vi "Get Config Variables.vi"(8 "error in (no error)":errorcluster, 10 "ReadBufferView":i32, 11 "LabVIEW Web Service Request":refnum<class "Web Request.lvclass">) -> (0 "error out":errorcluster, 3 "LabVIEW Web Service Request out":refnum<class "Web Request.lvclass">)   [LabVIEW 2018]
doc: "This VI sets all of the ESP variables for a single contact so it can be output from an ESP script."
uses:
  <vilib>/wsapi/Web Request.lvclass
  subvis/i32 to dec string small.vi
  CAEN globals.vi
  subvis/dbl to fr string small.vi
  <vilib>/wsapi/class/subVIs/Set Many String ESP Variables.vi
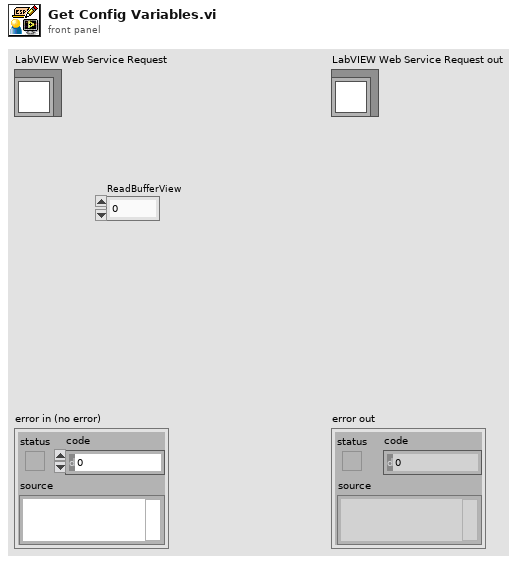
[diagram p1: front panel]
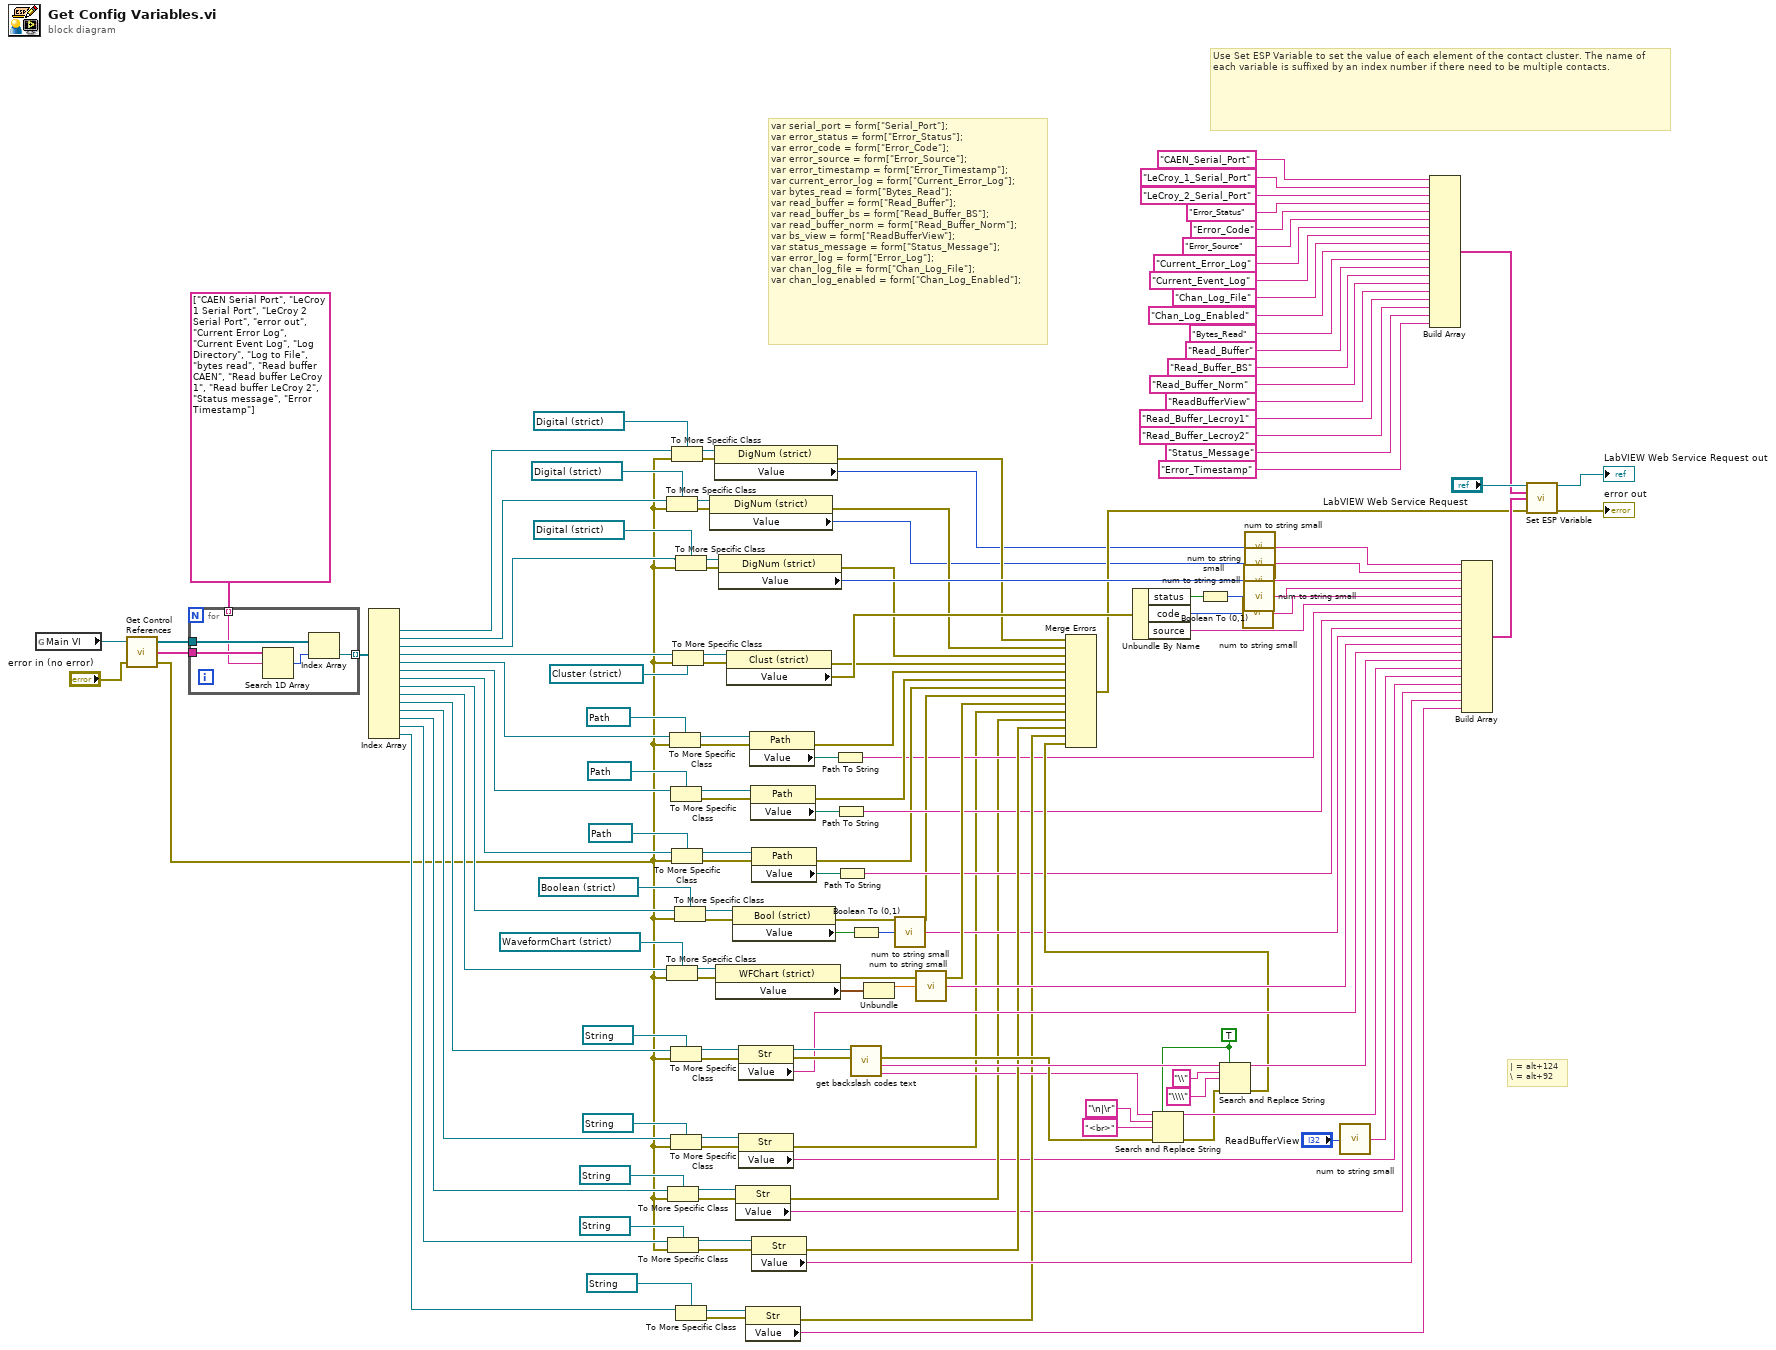
[diagram p0: block diagram]
diagram:
  w66 = TRUE ("replace all? (F)")
  # "| = alt+124\n\\ = alt+92"
  # "var serial_port = form[\"Serial_Port\"];\nvar error_status = form[\"Error_Status\"];\nvar error_code = form[\"Error_Code\"];\nvar error_source = form[\"Error_Source\"];\nvar error_timestamp = form[\"Error_Timestamp\"];\nvar current_error_log = form[\"Current_Error_Log\"];\nvar bytes_read = form[\"Bytes_Read\"];\nvar read_buffer = form[\"Read_Buffer\"];\nvar read_buffer_bs = form[\"Read_Buffer_BS\"];\nvar read_buffer_norm = form[\"Read_Buffer_Norm\"];\nvar bs_view = form[\"ReadBufferView\"];\nvar status_message = form[\"Status_Message\"];\nvar error_log = form[\"Error_Log\"];\nvar chan_log_file = form[\"Chan_Log_File\"];\nvar chan_log_enabled = form[\"Chan_Log_Enabled\"];"
  # "Use Set ESP Variable to set the value of each element of the contact cluster. The name of each variable is suffixed by an index number if there need to be multiple contacts."
  n1 = global read "CAEN globals.vi" "Main VI"() -> (w134:refnum<vi>)
  n2 = call "Get Control References.vi"("error in"="error in (no error)", "This vi"=w134) -> ("error out"=w3:errorcluster, "Control Names"=w133:string[], "Controls[]"=w132:refnum<vi>[])  [unwired: 1 in]
  n3 = for {
    tunnel: w133 -> [w152]
    tunnel: w132 -> [w150]
    tunnel: [w149] -> w124 mode=indexing
    tunnel: string[] ["CAEN Serial Port", "LeCroy 1 Serial Port", "LeCroy 2 Serial Port", "error out", "Current Error Log", "Current Event Log", "Log Directory", "Log to File", "bytes read", "Read buffer CAEN", "Read buffer LeCroy 1", "Read buffer LeCroy 2", "Status message", "Error Timestamp"] ("Control Names") -> [w148] mode=indexing
    n4 = Search 1D Array(1D array=w152, element=w148) -> (index of element=w151:i32)  [unwired: 1 in]
    n5 = Index Array(array=w150, index=w151) -> (element=w149:refnum<vi>)
  }
  n6 = Index Array(array=w124) -> (element #1=w18:refnum<vi>, element #2=w19:refnum<vi>, element #3=w122:refnum<vi>, element #4=w116:refnum<vi>, element #5=w112:refnum<vi>, element #6=w51:refnum<vi>, element #7=w44:refnum<vi>, element #8=w40:refnum<vi>, element #9=w38:refnum<vi>, element #10=w37:refnum<vi>, element #11=w4:refnum<vi>, element #12=w5:refnum<vi>, element #13=w6:refnum<vi>, element #14=w7:refnum<vi>)  [unwired: 14 in]
  n7 = To More Specific Class(target class=refnum<vi> refnum ("code"), reference=w19, error in=w3) -> (specific class reference=w30:refnum<vi>, error out=w29:errorcluster)
  n8 = To More Specific Class(target class=refnum<vi> refnum ("bytes read 2"), reference=w38, error in=w3) -> (specific class reference=w104:refnum<vi>, error out=w103:errorcluster)
  n9 = To More Specific Class(target class=refnum<vi> refnum ("Label.Text"), reference=w5, error in=w3) -> (specific class reference=w13:refnum<vi>, error out=w14:errorcluster)
  n10 = To More Specific Class(target class=refnum<vi> refnum ("Label.Text"), reference=w6, error in=w3) -> (specific class reference=w97:refnum<vi>, error out=w96:errorcluster)
  n11 = To More Specific Class(target class=refnum<vi> refnum ("Error Log Directory"), reference=w112, error in=w3) -> (specific class reference=w109:refnum<vi>, error out=w110:errorcluster)
  n12 = To More Specific Class(target class=refnum<vi> refnum ("Error Log Directory"), reference=w51) -> (specific class reference=w55:refnum<vi>, error out=w54:errorcluster)  [unwired: 1 in]
  n13 = To More Specific Class(target class=refnum<vi> refnum ("Label.Text"), reference=w37, error in=w3) -> (specific class reference=w106:refnum<vi>, error out=w107:errorcluster)
  n14 = To More Specific Class(target class=refnum<vi> refnum ("Label.Text"), reference=w4, error in=w3) -> (specific class reference=w16:refnum<vi>, error out=w15:errorcluster)
  n15 = To More Specific Class(target class=refnum<vi> refnum ("code"), reference=w18, error in=w3) -> (specific class reference=w27:refnum<vi>, error out=w28:errorcluster)
  n16 = To More Specific Class(target class=refnum<vi> refnum ("Error Log Directory"), reference=w44, error in=w3) -> (specific class reference=w46:refnum<vi>, error out=w47:errorcluster)
  n17 = To More Specific Class(target class=refnum<vi> refnum ("error in (no error)"), reference=w116, error in=w3) -> (specific class reference=w115:refnum<vi>, error out=w117:errorcluster)
  n18 = To More Specific Class(target class=refnum<vi> refnum ("replace all? (F)"), reference=w40, error in=w3) -> (specific class reference=w74:refnum<vi>, error out=w75:errorcluster)
  n19 = To More Specific Class(target class=refnum<vi> refnum ("code"), reference=w122, error in=w3) -> (specific class reference=w121:refnum<vi>, error out=w123:errorcluster)
  n20 = To More Specific Class(target class=refnum<vi> refnum ("Label.Text"), reference=w7) -> (specific class reference=w62:refnum<vi>, error out=w63:errorcluster)  [unwired: 1 in]
  n21 = property class="DigNum (strict)"(reference=w30, error in=w29) -> (error out=w24:errorcluster, "Value"=w21:i32)  [unwired: 1 out]
  n22 = property class="DigNum (strict)"(reference=w27, error in=w28) -> (error out=w25:errorcluster, "Value"=w20:i32)  [unwired: 1 out]
  n23 = property class="WFChart (strict)"(reference=w104, error in=w103) -> (error out=w52:errorcluster, "Value"=w101:cluster{dbl, "element":i32})  [unwired: 1 out]
  n24 = property class="DigNum (strict)"(reference=w121, error in=w123) -> (error out=w94:errorcluster, "Value"=w120:i32)  [unwired: 1 out]
  n25 = property class="Clust (strict)"(reference=w115, error in=w117) -> (error out=w93:errorcluster, "Value"=w113:errorcluster)  [unwired: 1 out]
  n26 = property class="Bool (strict)"(reference=w74, error in=w75) -> (error out=w41:errorcluster, "Value"=w72:bool)  [unwired: 1 out]
  n27 = property class="Str"(reference=w13, error in=w14) -> (error out=w10:errorcluster, "Value"=w8:string)  [unwired: 1 out]
  n28 = property class="Str"(reference=w106, error in=w107) -> (reference out=w87:refnum<vi>, error out=w86:errorcluster, "Value"=w80:string)
  n29 = property class="Str"(reference=w16, error in=w15) -> (error out=w11:errorcluster, "Value"=w9:string)  [unwired: 1 out]
  n30 = property class="Str"(reference=w62, error in=w63) -> (error out=w60:errorcluster, "Value"=w34:string)  [unwired: 1 out]
  n31 = property class="Path"(reference=w109, error in=w110) -> (error out=w92:errorcluster, "Value"=w108:path)  [unwired: 1 out]
  n32 = property class="Path"(reference=w55, error in=w54) -> (error out=w49:errorcluster, "Value"=w56:path)  [unwired: 1 out]
  n33 = property class="Path"(reference=w46, error in=w47) -> (error out=w42:errorcluster, "Value"=w45:path)  [unwired: 1 out]
  n34 = property class="Str"(reference=w97, error in=w96) -> (error out=w69:errorcluster, "Value"=w95:string)  [unwired: 1 out]
  n35 = Path To String(path=w108) -> (string=w35:string)
  n36 = Path To String(path=w56) -> (string=w50:string)
  n37 = Path To String(path=w45) -> (string=w43:string)
  n38 = Boolean To (0,1)(Boolean=w72) -> (0, 1=w71:i16)
  n39 = call "get backslash codes text.vi"("error in (no error)"=w86, "String in"=w87) -> ("normal text"=w65:string, "'\\' codes text"=w79:string, "error out"=w70:errorcluster)  [unwired: 6 in, 1 out]
  n40 = Unbundle(w101) -> (w99:dbl)  [unwired: 1 out]
  n41 = call-poly "num to string small.vi"("number"=w71) -> ("String"=w39:string)  [unwired: 14 in]
  n42 = call-poly "num to string small.vi"("number"=w99) -> ("String"=w100:string)  [unwired: 14 in]
  n43 = Unbundle By Name(w113) -> ("status"=w131:bool, "code"=w126:i32, "source"=w125:string)
  n44 = Search and Replace String(replace all?=w66, input string=w65, search string="\n|\r", replace string="<br>" ("replace string (\"\")"), error in=w70) -> (result string=w83:string, error out=w68:errorcluster)  [unwired: 3 in, 2 out]
  n45 = Boolean To (0,1)(Boolean=w131) -> (0, 1=w144:i16)
  n46 = Search and Replace String(replace all?=w66, input string=w79, search string="\\", replace string="\\\\" ("search string"), error in=w68) -> (result string=w76:string, error out=w67:errorcluster)  [unwired: 3 in, 2 out]
  n47 = Merge Errors(w25, w24, w94, w93, w92, w49, w42, w41, w52, w11, w10, w69, w60, w67) -> (w91:errorcluster)
  n48 = call-poly "num to string small.vi"("number"=w126) -> ("String"=w127:string)  [unwired: 14 in]
  n49 = call-poly "num to string small.vi"("number"=w120) -> ("String"=w118:string)  [unwired: 14 in]
  n50 = call-poly "num to string small.vi"("number"=w144) -> ("String"=w130:string)  [unwired: 14 in]
  n51 = call-poly "num to string small.vi"("number"=w20) -> ("String"=w22:string)  [unwired: 14 in]
  n52 = call-poly "num to string small.vi"("number"=w21) -> ("String"=w23:string)  [unwired: 14 in]
  n53 = call-poly "num to string small.vi"("number"="ReadBufferView") -> ("String"=w81:string)  [unwired: 14 in]
  n54 = Build Array("CAEN_Serial_Port" ("string"), "LeCroy_1_Serial_Port" ("string"), "LeCroy_2_Serial_Port" ("string"), "Error_Status" ("string"), "Error_Code" ("string"), "Error_Source" ("string"), "Current_Error_Log" ("string"), "Current_Event_Log" ("string"), "Chan_Log_File" ("string"), "Chan_Log_Enabled" ("string"), "Bytes_Read" ("string"), "Read_Buffer" ("string"), "Read_Buffer_BS" ("string"), "Read_Buffer_Norm" ("string"), "ReadBufferView" ("string"), "Read_Buffer_Lecroy1" ("string"), "Read_Buffer_Lecroy2" ("string"), "Status_Message" ("string"), "Error_Timestamp" ("string")) -> (w146:string[])
  n55 = Build Array(w22, w23, w118, w130, w127, w125, w35, w50, w43, w39, w100, w80, w76, w83, w81, w9, w8, w95, w34) -> (w145:string[])
  n56 = call-poly <vilib>:"Set ESP Variable.vi"("LabVIEW Web Service Request"="LabVIEW Web Service Request", "keys"=w146, "values"=w145, "error in (no error)"=w91) -> ("LabVIEW Web Service Request out"=→"LabVIEW Web Service Request out":refnum<class "Web Request.lvclass">, "error out"=→"error out":errorcluster)  [unwired: 10 in]
